vi "sample clock continous.vi"(8 "error in (no error)":errorcluster, 9 "rate":dbl=1000.0, 10 "number of samples":i32=1000, 11 "Refnum in":refnum<k21>) -> (0 "error out":errorcluster, 3 "Refnum out":refnum<k21>)   [LabVIEW 2018]
uses:
  <vilib>/DAQmx/configure/timing.llb/DAQmx Timing (Sample Clock).vi
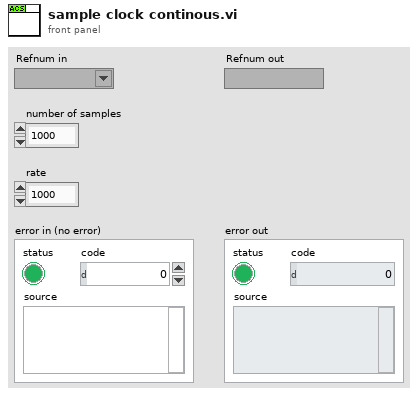
[diagram p1: front panel]
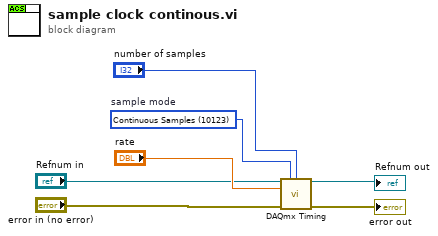
[diagram p0: block diagram]
diagram:
  w4 = 10123 items=["Finite Samples"=10178, "Continuous Samples"=10123, "Hardware Timed Single Point"=12522]  # sample mode
  n1 = call-poly <vilib>:"DAQmx Timing.vi"("task/channels in"="Refnum in", "sample mode"=w4, "samples per channel"="number of samples", "rate"="rate", "error in"="error in (no error)") -> ("task out"=→"Refnum out":refnum<k21>, "error out"=→"error out":errorcluster)  [unwired: 9 in]
